vi "ButtonCycle.vi"(9 "MaxNum":dbl, 10 "FlashInput":bool) -> (2 "CycleNumber":dbl)   [LabVIEW 2020]
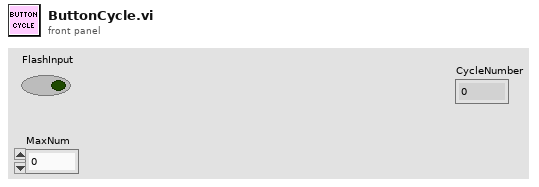
[diagram p1: front panel]
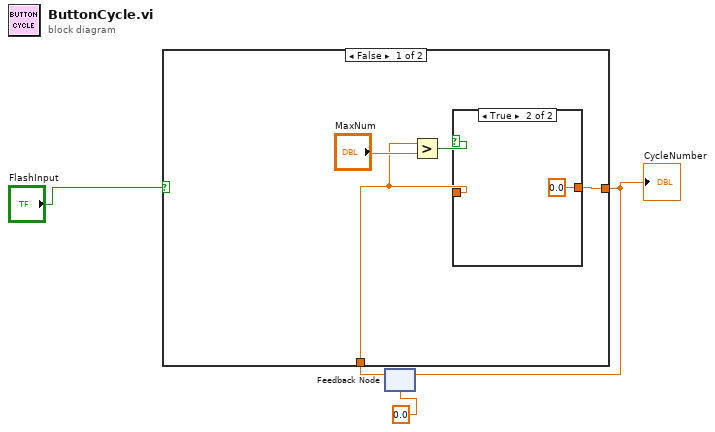
[diagram p0: block diagram]
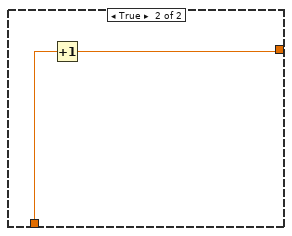
[diagram p3: hidden frame]
diagram:
  n1 = feedback #1(0.0) -> (w2:dbl)
  n2 = case shown="False" "FlashInput" {
    tunnel: [w6 w12] -> w3
    tunnel: w2 -> [w5 w11]
    frame False {
      n3 = Greater?(x=w5, y="MaxNum") -> (0:w7:bool)
      n4 = case shown="True" w7 {
        tunnel: [w9 0.0] -> w6
        tunnel: w5 -> [w9 _]
        frame False {
        }
        frame True {
        }
      }
    }
    frame True {
      n5 = Increment(x=w11) -> (x+1=w12:dbl)
    }
  }
  "CycleNumber" <- w3
  n6 = feedback-in #1(w3) -> ()
